vi "Parameters.vi"(8 "error in (no error)":errorcluster, 11 "Template Test Case In":refnum<class "API Pass Output.lvclass">) -> (0 "error out":errorcluster, 2 "Parameters":T1(array[cluster]))   [LabVIEW 2020, in "API Pass Output.lvclass"]
doc: "This VI defines the parameters used for execution. When LUnit runs the test case, it will run it once for every parameter in the array and collect the results.\n\nDuring test execution, the parameters are available in the class wire within the test VI."
uses:
  API Pass Output.lvclass
  API Pass Output.lvclass/API Pass Output.ctl
  <vilib>/Astemes/LUnit Parameterized/Parameterized Test Case/Parameterized Test Case.lvclass
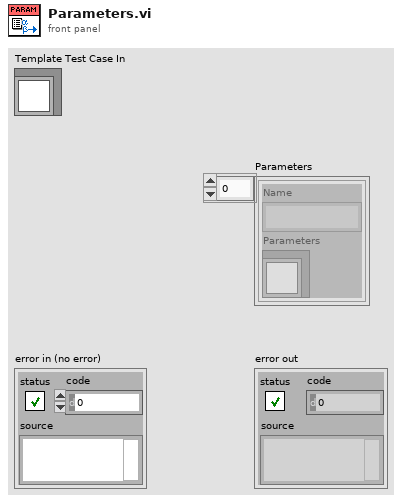
[diagram p1: front panel]
types:
  T1 = cluster{"Name":string, "Parameters":refnum<class "Parameterized Test Case.lvclass">}[]
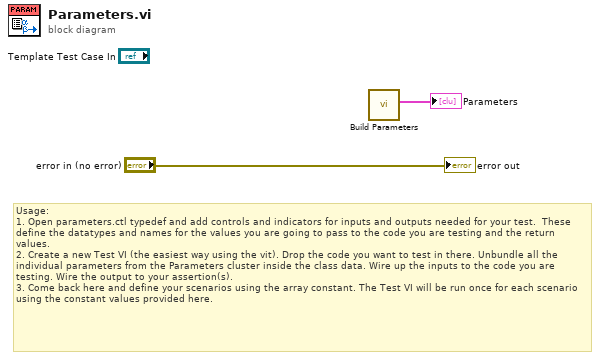
[diagram p0: block diagram]
diagram:
  # "Usage:\n1. Open parameters.ctl typedef and add controls and indicators for inputs and outputs needed for your test.  These define the datatypes and names for the values you are going to pass to the code you are testing and the return values.\n2. Create a new Test VI (the easiest way using the vit). Drop the code you want to test in there. Unbundle all the individual parameters from the Parameters cluster inside the class data. Wire up the inputs to the code you are testing. Wire the output to your assertion(s).\n3. Come back here and define your scenarios using the array constant. The Test VI will be run once for each scenario using the constant values provided here."
  n1 = call "Build Parameters.vi"() -> ("Scenarios"=→"Parameters":T1)  [unwired: 11 in]
  "error out" <- "error in (no error)"
